vi "QtoMtoQ.vi"(4 "Pressure":dbl=1000.0 caption="Pressure (mBar)" format="%#.1fmBar", 5 "Temperature":dbl caption="Temp (C)" format="%.1fC", 6 "Mdot in (g/min)":dbl, 7 "Q in (l/min)":dbl, 9 "Gas":T1="Air") -> (0 "Q out (l/min)":dbl, 1 "Mdot out (g/min)":dbl, 3 "Density (kg/m^3)(= g/l)":dbl)   [LabVIEW 2021]
uses:
  Controls/GasCombo.ctl
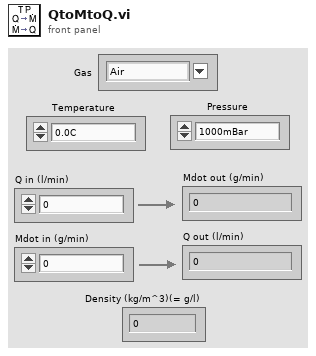
[diagram p1: front panel]
types:
  T1 = typedef "GasCombo.ctl" = string
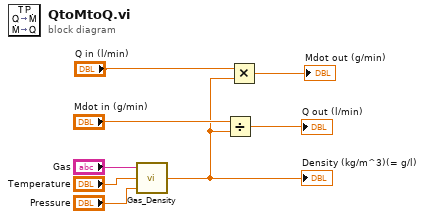
[diagram p0: block diagram]
diagram:
  n1 = call "Gas_Density.vi"("Pressure (mbar)"="Pressure", "Temperature (C)"="Temperature", "Gas"="Gas") -> ("Density (kg/m^3) (= g/l)"=w1:dbl)
  "Density (kg/m^3)(= g/l)" <- w1
  n2 = Divide(x="Mdot in (g/min)", y=w1) -> (x/y=→"Q out (l/min)":dbl)
  n3 = Multiply(x="Q in (l/min)", y=w1) -> (x*y=→"Mdot out (g/min)":dbl)
